vi "9871_EPICS_FPGA_Main.vi"() -> ()   [LabVIEW 2020]
uses:
  <vilib>/rvi/Emulation/niFpgaGetClockAttributes.vi
  <vilib>/rvi/Emulation/niFpgaSctlEmulationGetInTimedLoop.vi
  <vilib>/rvi/Emulation/niFpgaEmulationReportErrorSimple.vi
  <vilib>/rvi/interface/RandomDataEmulation/niFpgaRandomDataHandleErrors.vi
  <vilib>/rvi/eio/common/nirviEmuTemplateMethod_errors.vi
  <vilib>/rvi/Emulation/niFpgaCriticalErrorInLSC.vi
  <vilib>/rvi/eio/common/nirviEmuTemplatePropertySet_errors.vi
  <vilib>/rvi/DataTransferAndStorage/Container/XNode/niFpgaContainer.xnode
  <vilib>/rvi/interface/RandomDataEmulation/nirviRandomDataFpgaReadWriteTemplate.vi
  <vilib>/eio/EIOMethodNode/EIOMethodNode.xnode
  <vilib>/eio/EIOPropertyNode/EIOPropertyNode.xnode
  <vilib>/LabVIEW Targets/FPGA/cRIO/shared/nicrio_ModuleControls/nicrio_cRIO-9871_BaudRateEnum.ctl
  <vilib>/LabVIEW Targets/FPGA/cRIO/shared/nicrio_ModuleControls/nicrio_cRIO-9871_DataBitsEnum.ctl
  <vilib>/LabVIEW Targets/FPGA/cRIO/shared/nicrio_ModuleControls/nicrio_cRIO-9871_FlowControlEnum.ctl
  <vilib>/LabVIEW Targets/FPGA/cRIO/shared/nicrio_ModuleControls/nicrio_cRIO-9871_ParityEnum.ctl
  <vilib>/LabVIEW Targets/FPGA/cRIO/shared/nicrio_ModuleControls/nicrio_cRIO-9871_StopBitsEnum.ctl
  <vilib>/rvi/eio/common/nirviEmuTemplatePropertyGet_errors.vi
  <vilib>/rvi/eio/common/nirviEmuTemplatePropertyGet_noerrors.vi
  <vilib>/rvi/eio/common/nirviEmuTemplatePropertySet_noerrors.vi
panel:
  out "P3ReadError":errorcluster
  out "RX3FIFOTOCount":u32
  out "RX3ErrorCount":u32
  out "P4ReadError":errorcluster
  out "RX4FIFOTOCount":u32
  out "RX4ErrorCount":u32
  out "P2ReadError":errorcluster
  out "RX2FIFOTOCount":u32
  out "RX2ErrorCount":u32
  out "RX1FIFOTOCount":u32
  out "RX1ErrorCount":u32
  out "TXTOCount":u32
  out "TXErrorCount":u32
  out "P1ReadError":errorcluster
  out "WriteError":errorcluster
  # "WRITE"
  # "READ"
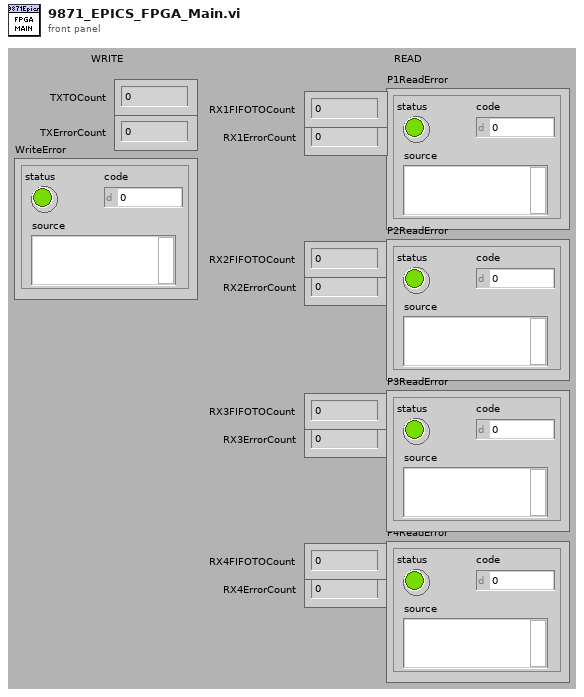
[diagram p1: front panel]
types:
  T1 = enum16{"TX Byte", "TX Clear", "Echo Request", "Parameter Change"}
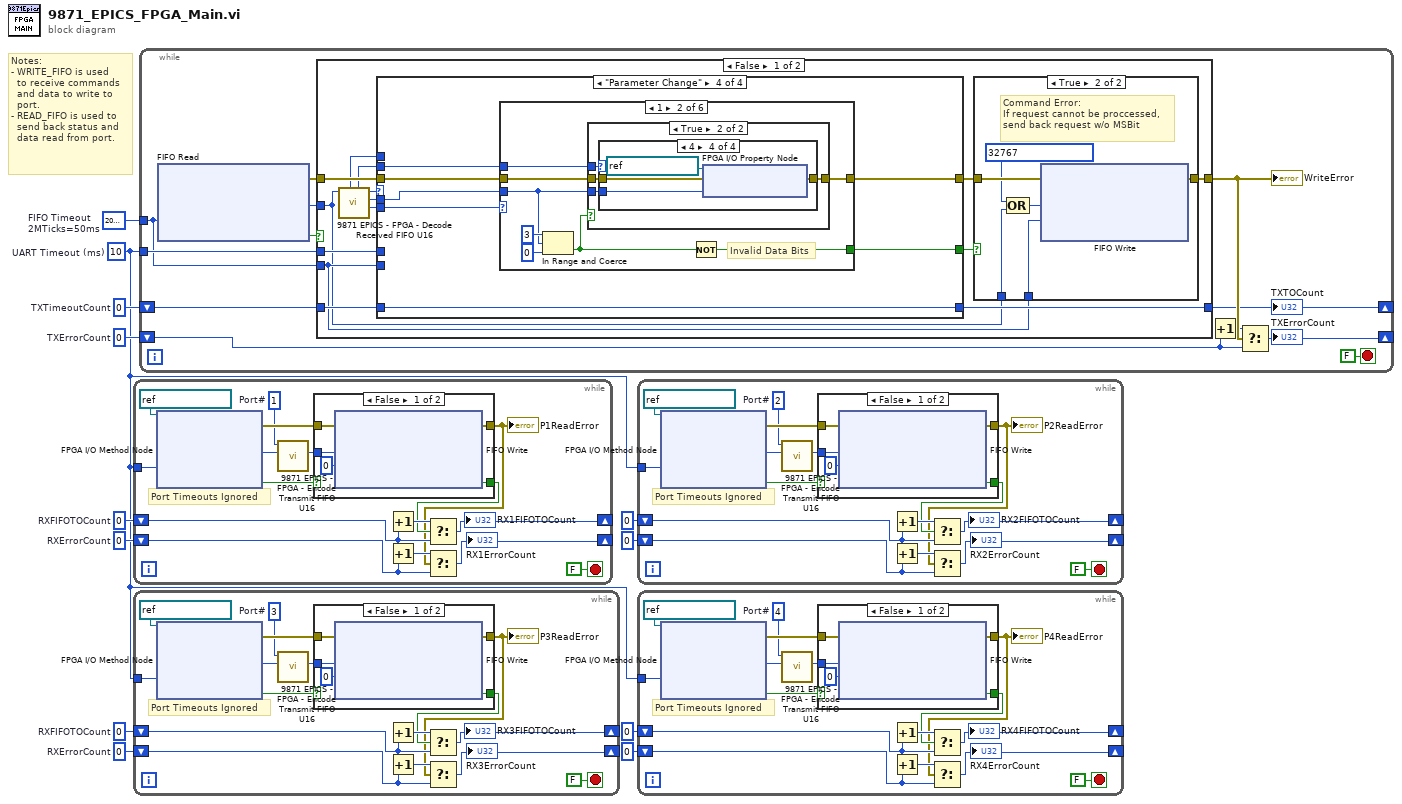
[diagram p0: block diagram]
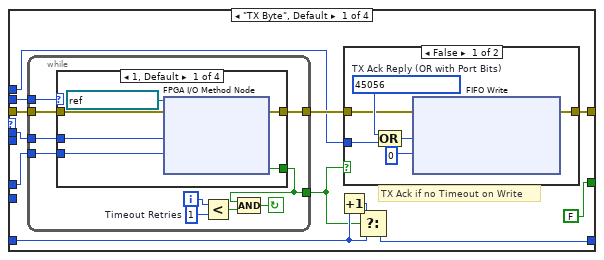
[diagram p6: hidden frame]
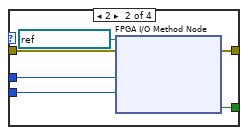
[diagram p8: hidden frame]
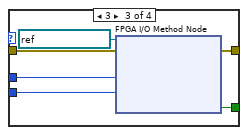
[diagram p9: hidden frame]
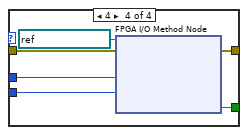
[diagram p10: hidden frame]
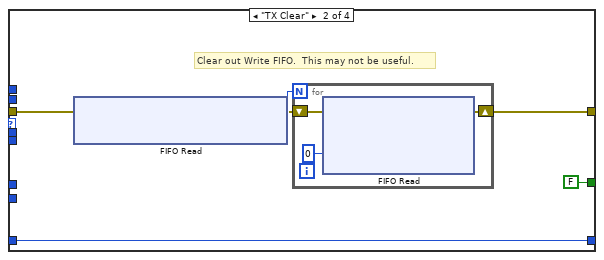
[diagram p11: hidden frame]
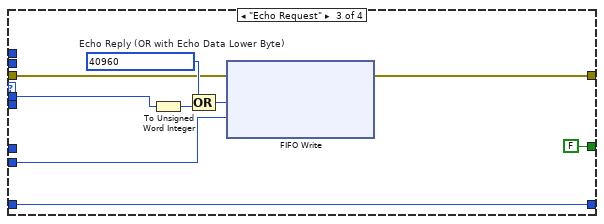
[diagram p12: hidden frame]
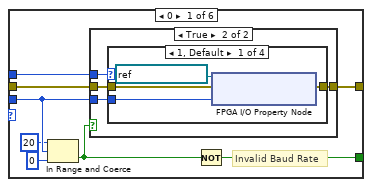
[diagram p13: hidden frame]
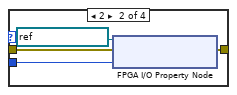
[diagram p15: hidden frame]
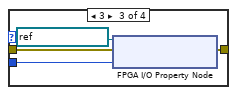
[diagram p16: hidden frame]
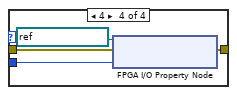
[diagram p17: hidden frame]
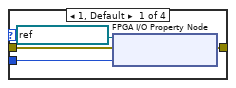
[diagram p19: hidden frame]
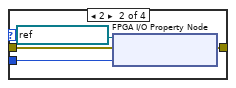
[diagram p20: hidden frame]
diagram:
  w3 = u32 0  # RXErrorCount
  w2 = u32 0  # RXFIFOTOCount
  w8 = u32 0  # RXErrorCount
  w9 = u32 0  # RXFIFOTOCount
  w10 = u32 0  # TXErrorCount
  w1 = 10  # UART Timeout (ms)
  w12 = 2000000  # FIFO Timeout 2MTicks=50ms
  w11 = u32 0  # TXTimeoutCount
  # "Notes:\n- WRITE_FIFO is used\n  to receive commands\n  and data to write to\n  port.\n- READ_FIFO is used to\n  send back status and\n  data read from port."
  n1 = while {
    tunnel: w1 -> [w26]
    shift-right: [w14] -> _
    shift-left: w9 -> [w18]
    shift-right: [w13] -> _
    shift-left: w8 -> [w15]
    stop <- FALSE stop-if-true
    w22 = u8 1  # Port#
    # "Port Timeouts Ignored"
    n2 = xnode "FPGA I/O Method Node"("FPGA I/O In"=refnum<k21> "Mod1\\Port1" ("cRIO I/O Device"), "Timeout (ms)"=w26) -> ("error out"=w24:errorcluster, "Data"=w23:u8, "Timed Out"=w25:bool)  [unwired: 1 in, 1 out]
    n3 = call "9871 EPICS - FPGA - Encode Transmit FIFO U16.vi"("Data Byte"=w23, "Port# (1-4)"=w22) -> ("U16 to Send to TX FIFO"=w21:u16)  [unwired: 9 in]
    n4 = case shown="False" w25 {
      tunnel: [w33 _] -> w19
      tunnel: w21 -> [w29 _]
      tunnel: [w31 w34] -> w16
      tunnel: w24 -> [w30 w34]
      frame False {
        n5 = xnode ("FIFO Write")("Element"=w29, "Timeout"=0, "error in (no error)"=w30) -> ("Timed Out?"=w33:bool, "error out"=w31:errorcluster)  [unwired: 1 in, 1 out]
      }
      frame True {
      }
    }
    "P1ReadError" <- w16
    n6 = Increment(x=w18) -> (x+1=w20:u32)
    n7 = Increment(x=w15) -> (x+1=w17:u32)
    n8 = Select(t=w20, s=w19, f=w18) -> (s? t:f=w14:u32)
    "RX1FIFOTOCount" <- w14
    n9 = Select(t=w17, s=w16, f=w15) -> (s? t:f=w13:u32)
    "RX1ErrorCount" <- w13
  }
  n10 = while {
    tunnel: w1 -> [w48]
    shift-right: [w36] -> _
    shift-left: w2 -> [w40]
    shift-right: [w35] -> _
    shift-left: w3 -> [w37]
    stop <- FALSE stop-if-true
    w44 = u8 3  # Port#
    # "Port Timeouts Ignored"
    n11 = xnode "FPGA I/O Method Node"("FPGA I/O In"=refnum<k21> "Mod1\\Port3" ("cRIO I/O Device"), "Timeout (ms)"=w48) -> ("error out"=w46:errorcluster, "Data"=w45:u8, "Timed Out"=w47:bool)  [unwired: 1 in, 1 out]
    n12 = call "9871 EPICS - FPGA - Encode Transmit FIFO U16.vi"("Data Byte"=w45, "Port# (1-4)"=w44) -> ("U16 to Send to TX FIFO"=w43:u16)  [unwired: 9 in]
    n13 = case shown="False" w47 {
      tunnel: [w55 _] -> w41
      tunnel: w43 -> [w51 _]
      tunnel: [w53 w56] -> w38
      tunnel: w46 -> [w52 w56]
      frame False {
        n14 = xnode ("FIFO Write")("Element"=w51, "Timeout"=0, "error in (no error)"=w52) -> ("Timed Out?"=w55:bool, "error out"=w53:errorcluster)  [unwired: 1 in, 1 out]
      }
      frame True {
      }
    }
    "P3ReadError" <- w38
    n15 = Increment(x=w40) -> (x+1=w42:u32)
    n16 = Increment(x=w37) -> (x+1=w39:u32)
    n17 = Select(t=w42, s=w41, f=w40) -> (s? t:f=w36:u32)
    "RX3FIFOTOCount" <- w36
    n18 = Select(t=w39, s=w38, f=w37) -> (s? t:f=w35:u32)
    "RX3ErrorCount" <- w35
  }
  n19 = while {
    shift-right: [w57] -> _
    shift-left: w11 -> [w64]
    tunnel: w12 -> [w62]
    tunnel: w1 -> [w63]
    shift-right: [w58] -> _
    shift-left: w10 -> [w59]
    stop <- FALSE stop-if-true
    n20 = xnode ("FIFO Read")("Timeout"=w62) -> ("Element"=w65:u16, "Timed Out?"=w66:bool, "error out"=w67:errorcluster)  [unwired: 2 in, 1 out]
    n21 = case shown="False" w66 {
      tunnel: [w72 w316] -> w61
      tunnel: w63 -> [w82 _]
      tunnel: w67 -> [w81 w316]
      tunnel: w65 -> [w70 _]
      tunnel: w64 -> [w78 w315]
      tunnel: [w77 w315] -> w57
      tunnel: w62 -> [w71 _]
      frame False {
        n22 = call "9871 EPICS - FPGA - Decode Received FIFO U16.vi"("U16"=w70) -> ("Parameter High Nibble Mid 4 bits  (xxNNNNxx xxxxxxxx)"=w74:u8, "Low Byte (xxxxxxxx NNNNNNNN)"=w79:u8, "Request Type"=w80:T1, "Port# (1-4)"=w76:u8, "Port Bits Only in U16"=w75:u16)  [unwired: 6 in]
        n23 = case shown="\"Parameter Change\"" w80 {
          tunnel: [w93 w144 w153 w162] -> w73
          tunnel: w82 -> [w101 _ _ _]
          tunnel: w81 -> [w98 w147 w154 w165]
          tunnel: w79 -> [w99 _ w159 w166]
          tunnel: w76 -> [w100 _ _ w163]
          tunnel: w78 -> [w96 w148 w160 w167]
          tunnel: [w97 w148 w160 w167] -> w77
          tunnel: w71 -> [_ _ w157 _]
          tunnel: w75 -> [w91 _ _ _]
          tunnel: w74 -> [_ _ _ w164]
          tunnel: [FALSE FALSE FALSE w161] -> w69
          frame "TX Byte", Default {
            # "TX Ack if no Timeout on Write"
            n24 = while {
              tunnel: w101 -> [w118]
              tunnel: [w112] -> w92
              tunnel: w100 -> [w117]
              tunnel: w99 -> [w116]
              tunnel: w98 -> [w111]
              tunnel: [w110] -> w94
              i -> [w115]
              stop <- w109 continue-if-true
              w114 = 1  # Timeout Retries
              n25 = case shown="1, Default" w117 {
                tunnel: w116 -> [w124 w130 w136 w142]
                tunnel: w118 -> [w123 w129 w135 w141]
                tunnel: [w122 w128 w134 w140] -> w112
                tunnel: w111 -> [w121 w127 w133 w139]
                tunnel: [w120 w126 w132 w138] -> w110
                frame 1, Default {
                  n26 = xnode "FPGA I/O Method Node"("error in"=w121, "FPGA I/O In"=refnum<k21> "Mod1\\Port1" ("cRIO I/O Device"), "Data"=w124, "Timeout (ms)"=w123) -> ("error out"=w120:errorcluster, "Timed Out"=w122:bool)  [unwired: 1 out]
                }
                frame 2 {
                  n27 = xnode "FPGA I/O Method Node"("error in"=w127, "FPGA I/O In"=refnum<k21> "Mod1\\Port2" ("cRIO I/O Device"), "Data"=w130, "Timeout (ms)"=w129) -> ("error out"=w126:errorcluster, "Timed Out"=w128:bool)  [unwired: 1 out]
                }
                frame 3 {
                  n28 = xnode "FPGA I/O Method Node"("error in"=w133, "FPGA I/O In"=refnum<k21> "Mod1\\Port3" ("cRIO I/O Device"), "Data"=w136, "Timeout (ms)"=w135) -> ("error out"=w132:errorcluster, "Timed Out"=w134:bool)  [unwired: 1 out]
                }
                frame 4 {
                  n29 = xnode "FPGA I/O Method Node"("error in"=w139, "FPGA I/O In"=refnum<k21> "Mod1\\Port4" ("cRIO I/O Device"), "Data"=w142, "Timeout (ms)"=w141) -> ("error out"=w138:errorcluster, "Timed Out"=w140:bool)  [unwired: 1 out]
                }
              }
              n30 = Less?(x=w115, y=w114) -> (x < y?=w113:bool)
              n31 = Compound Arithmetic op=AND(w112, w113) -> (w109:bool)
            }
            n32 = Increment(x=w96) -> (x+1=w95:u32)
            n33 = case shown="False" w92 {
              tunnel: w94 -> [w105 w108]
              tunnel: [w104 w108] -> w93
              tunnel: w91 -> [w103 _]
              frame False {
                w106 = u16 45056  # TX Ack Reply (OR with Port Bits)
                n34 = Compound Arithmetic op=OR(w106, w103) -> (w107:u16)
                n35 = xnode ("FIFO Write")("Element"=w107, "Timeout"=0, "error in (no error)"=w105) -> ("error out"=w104:errorcluster)  [unwired: 1 in, 2 out]
              }
              frame True {
              }
            }
            n36 = Select(t=w95, s=w92, f=w96) -> (s? t:f=w97:u32)
          }
          frame "TX Clear" {
            # "Clear out Write FIFO.  This may not be useful."
            n37 = xnode ("FIFO Read")("error in (no error)"=w147) -> ("Number of Elements to Read"=w146:u32, "error out"=w145:errorcluster)  [unwired: 1 in, 1 out]
            n38 = for {
              N: w146 -> [_]
              shift-right: [w150] -> w144
              shift-left: w145 -> [w151]
              n39 = xnode ("FIFO Read")("Timeout"=0, "error in (no error)"=w151) -> ("error out"=w150:errorcluster)  [unwired: 1 in, 3 out]
            }
          }
          frame "Echo Request" {
            w156 = u16 40960  # Echo Reply (OR with Echo Data Lower Byte)
            n40 = To Unsigned Word Integer(number=w159) -> (unsigned 16bit integer=w158:u16)
            n41 = Compound Arithmetic op=OR(w156, w158) -> (w155:u16)
            n42 = xnode ("FIFO Write")("Element"=w155, "Timeout"=w157, "error in (no error)"=w154) -> ("error out"=w153:errorcluster)  [unwired: 1 in, 2 out]
          }
          frame "Parameter Change" {
            n43 = case shown="1" w164 {
              tunnel: w166 -> [w172 w199 w228 w256 w286 _]
              tunnel: w165 -> [w175 w204 w233 w262 w291 w314]
              tunnel: [w174 w203 w232 w261 w290 w314] -> w162
              tunnel: [w168 w198 w227 w257 w285 w313] -> w161
              tunnel: w163 -> [w173 w202 w231 w260 w289 _]
              frame 0 {
                # "Invalid Baud Rate"
                n44 = In Range and Coerce(upper limit=u8 20, x=w172, lower limit=u8 0) -> (In Range?=w169:bool)  [unwired: 1 out]
                n45 = case shown="True" w169 {
                  tunnel: w175 -> [w176 w180]
                  tunnel: [w176 w179] -> w174
                  tunnel: w173 -> [_ w178]
                  tunnel: w172 -> [_ w177]
                  frame False {
                  }
                  frame True {
                    n46 = case shown="1, Default" w178 {
                      tunnel: w177 -> [w183 w187 w191 w195]
                      tunnel: w180 -> [w182 w186 w190 w194]
                      tunnel: [w181 w185 w189 w193] -> w179
                      frame 1, Default {
                        n47 = xnode "FPGA I/O Property Node"("error in"=w182, "FPGA I/O In"=refnum<k21> "Mod1\\Port1" ("cRIO I/O Device"), "Baud Rate"=w183) -> ("error out"=w181:errorcluster)  [unwired: 1 out]
                      }
                      frame 2 {
                        n48 = xnode "FPGA I/O Property Node"("error in"=w186, "FPGA I/O In"=refnum<k21> "Mod1\\Port2" ("cRIO I/O Device"), "Baud Rate"=w187) -> ("error out"=w185:errorcluster)  [unwired: 1 out]
                      }
                      frame 3 {
                        n49 = xnode "FPGA I/O Property Node"("error in"=w190, "FPGA I/O In"=refnum<k21> "Mod1\\Port3" ("cRIO I/O Device"), "Baud Rate"=w191) -> ("error out"=w189:errorcluster)  [unwired: 1 out]
                      }
                      frame 4 {
                        n50 = xnode "FPGA I/O Property Node"("error in"=w194, "FPGA I/O In"=refnum<k21> "Mod1\\Port4" ("cRIO I/O Device"), "Baud Rate"=w195) -> ("error out"=w193:errorcluster)  [unwired: 1 out]
                      }
                    }
                  }
                }
                n51 = Not(x=w169) -> (.not. x?=w168:bool)
              }
              frame 1 {
                # "Invalid Data Bits"
                n52 = In Range and Coerce(upper limit=u8 3, x=w199, lower limit=u8 0) -> (In Range?=w197:bool)  [unwired: 1 out]
                n53 = case shown="True" w197 {
                  tunnel: w204 -> [w205 w209]
                  tunnel: [w205 w208] -> w203
                  tunnel: w202 -> [_ w207]
                  tunnel: w199 -> [_ w206]
                  frame False {
                  }
                  frame True {
                    n54 = case shown="4" w207 {
                      tunnel: w206 -> [w212 w216 w220 w224]
                      tunnel: w209 -> [w211 w215 w219 w223]
                      tunnel: [w210 w214 w218 w222] -> w208
                      frame 1, Default {
                        n55 = xnode "FPGA I/O Property Node"("error in"=w211, "FPGA I/O In"=refnum<k21> "Mod1\\Port1" ("cRIO I/O Device"), "Data Bits"=w212) -> ("error out"=w210:errorcluster)  [unwired: 1 out]
                      }
                      frame 2 {
                        n56 = xnode "FPGA I/O Property Node"("error in"=w215, "FPGA I/O In"=refnum<k21> "Mod1\\Port2" ("cRIO I/O Device"), "Data Bits"=w216) -> ("error out"=w214:errorcluster)  [unwired: 1 out]
                      }
                      frame 3 {
                        n57 = xnode "FPGA I/O Property Node"("error in"=w219, "FPGA I/O In"=refnum<k21> "Mod1\\Port3" ("cRIO I/O Device"), "Data Bits"=w220) -> ("error out"=w218:errorcluster)  [unwired: 1 out]
                      }
                      frame 4 {
                        n58 = xnode "FPGA I/O Property Node"("error in"=w223, "FPGA I/O In"=refnum<k21> "Mod1\\Port4" ("cRIO I/O Device"), "Data Bits"=w224) -> ("error out"=w222:errorcluster)  [unwired: 1 out]
                      }
                    }
                  }
                }
                n59 = Not(x=w197) -> (.not. x?=w198:bool)
              }
              frame 2 {
                # "Invalid Flow Control"
                n60 = In Range and Coerce(upper limit=u8 2, x=w228, lower limit=u8 0) -> (In Range?=w226:bool)  [unwired: 1 out]
                n61 = case shown="True" w226 {
                  tunnel: w233 -> [w234 w238]
                  tunnel: [w234 w237] -> w232
                  tunnel: w231 -> [_ w236]
                  tunnel: w228 -> [_ w235]
                  frame False {
                  }
                  frame True {
                    n62 = case shown="1, Default" w236 {
                      tunnel: w235 -> [w241 w245 w249 w253]
                      tunnel: w238 -> [w240 w244 w248 w252]
                      tunnel: [w239 w243 w247 w251] -> w237
                      frame 1, Default {
                        n63 = xnode "FPGA I/O Property Node"("error in"=w240, "FPGA I/O In"=refnum<k21> "Mod1\\Port1" ("cRIO I/O Device"), "Flow Control"=w241) -> ("error out"=w239:errorcluster)  [unwired: 1 out]
                      }
                      frame 2 {
                        n64 = xnode "FPGA I/O Property Node"("error in"=w244, "FPGA I/O In"=refnum<k21> "Mod1\\Port2" ("cRIO I/O Device"), "Flow Control"=w245) -> ("error out"=w243:errorcluster)  [unwired: 1 out]
                      }
                      frame 3 {
                        n65 = xnode "FPGA I/O Property Node"("error in"=w248, "FPGA I/O In"=refnum<k21> "Mod1\\Port3" ("cRIO I/O Device"), "Flow Control"=w249) -> ("error out"=w247:errorcluster)  [unwired: 1 out]
                      }
                      frame 4 {
                        n66 = xnode "FPGA I/O Property Node"("error in"=w252, "FPGA I/O In"=refnum<k21> "Mod1\\Port4" ("cRIO I/O Device"), "Flow Control"=w253) -> ("error out"=w251:errorcluster)  [unwired: 1 out]
                      }
                    }
                  }
                }
                n67 = Not(x=w226) -> (.not. x?=w227:bool)
              }
              frame 3 {
                # "Invalid Parity"
                n68 = In Range and Coerce(upper limit=u8 4, x=w256, lower limit=u8 0) -> (In Range?=w255:bool)  [unwired: 1 out]
                n69 = case shown="True" w255 {
                  tunnel: w262 -> [w263 w267]
                  tunnel: [w263 w266] -> w261
                  tunnel: w260 -> [_ w265]
                  tunnel: w256 -> [_ w264]
                  frame False {
                  }
                  frame True {
                    n70 = case shown="4" w265 {
                      tunnel: w264 -> [w270 w274 w278 w282]
                      tunnel: w267 -> [w269 w273 w277 w281]
                      tunnel: [w268 w272 w276 w280] -> w266
                      frame 1, Default {
                        n71 = xnode "FPGA I/O Property Node"("error in"=w269, "FPGA I/O In"=refnum<k21> "Mod1\\Port1" ("cRIO I/O Device"), "Parity"=w270) -> ("error out"=w268:errorcluster)  [unwired: 1 out]
                      }
                      frame 2 {
                        n72 = xnode "FPGA I/O Property Node"("error in"=w273, "FPGA I/O In"=refnum<k21> "Mod1\\Port2" ("cRIO I/O Device"), "Parity"=w274) -> ("error out"=w272:errorcluster)  [unwired: 1 out]
                      }
                      frame 3 {
                        n73 = xnode "FPGA I/O Property Node"("error in"=w277, "FPGA I/O In"=refnum<k21> "Mod1\\Port3" ("cRIO I/O Device"), "Parity"=w278) -> ("error out"=w276:errorcluster)  [unwired: 1 out]
                      }
                      frame 4 {
                        n74 = xnode "FPGA I/O Property Node"("error in"=w281, "FPGA I/O In"=refnum<k21> "Mod1\\Port4" ("cRIO I/O Device"), "Parity"=w282) -> ("error out"=w280:errorcluster)  [unwired: 1 out]
                      }
                    }
                  }
                }
                n75 = Not(x=w255) -> (.not. x?=w257:bool)
              }
              frame 4 {
                # "Invalid Stop Bits"
                n76 = In Range and Coerce(upper limit=u8 2, x=w286, lower limit=u8 0) -> (In Range?=w284:bool)  [unwired: 1 out]
                n77 = case shown="True" w284 {
                  tunnel: w291 -> [w292 w296]
                  tunnel: [w292 w295] -> w290
                  tunnel: w289 -> [_ w294]
                  tunnel: w286 -> [_ w293]
                  frame False {
                  }
                  frame True {
                    n78 = case shown="4" w294 {
                      tunnel: w293 -> [w299 w303 w307 w311]
                      tunnel: w296 -> [w298 w302 w306 w310]
                      tunnel: [w297 w301 w305 w309] -> w295
                      frame 1, Default {
                        n79 = xnode "FPGA I/O Property Node"("error in"=w298, "FPGA I/O In"=refnum<k21> "Mod1\\Port1" ("cRIO I/O Device"), "Stop Bits"=w299) -> ("error out"=w297:errorcluster)  [unwired: 1 out]
                      }
                      frame 2 {
                        n80 = xnode "FPGA I/O Property Node"("error in"=w302, "FPGA I/O In"=refnum<k21> "Mod1\\Port2" ("cRIO I/O Device"), "Stop Bits"=w303) -> ("error out"=w301:errorcluster)  [unwired: 1 out]
                      }
                      frame 3 {
                        n81 = xnode "FPGA I/O Property Node"("error in"=w306, "FPGA I/O In"=refnum<k21> "Mod1\\Port3" ("cRIO I/O Device"), "Stop Bits"=w307) -> ("error out"=w305:errorcluster)  [unwired: 1 out]
                      }
                      frame 4 {
                        n82 = xnode "FPGA I/O Property Node"("error in"=w310, "FPGA I/O In"=refnum<k21> "Mod1\\Port4" ("cRIO I/O Device"), "Stop Bits"=w311) -> ("error out"=w309:errorcluster)  [unwired: 1 out]
                      }
                    }
                  }
                }
                n83 = Not(x=w284) -> (.not. x?=w285:bool)
              }
              frame 5.. {
                w313 = TRUE  # Invalid UART Parameter ID
              }
            }
          }
        }
        n84 = case shown="True" w69 {
          tunnel: w73 -> [w83 w88]
          tunnel: [w83 w87] -> w72
          tunnel: w71 -> [_ w86]
          tunnel: w70 -> [_ w85]
          frame False {
          }
          frame True {
            # "Command Error:\nIf request cannot be proccessed,\nsend back request w/o MSBit"
            n85 = Compound Arithmetic op=OR(u16 32767, w85) -> (w89:u16)
            n86 = xnode ("FIFO Write")("Element"=w89, "Timeout"=w86, "error in (no error)"=w88) -> ("error out"=w87:errorcluster)  [unwired: 1 in, 2 out]
          }
        }
      }
      frame True {
      }
    }
    "WriteError" <- w61
    "TXTOCount" <- w57
    n87 = Increment(x=w59) -> (x+1=w60:u32)
    n88 = Select(t=w60, s=w61, f=w59) -> (s? t:f=w58:u32)
    "TXErrorCount" <- w58
  }
  n89 = while {
    tunnel: w1 -> [w330]
    shift-right: [w318] -> _
    shift-left: u32 0 ("RXFIFOTOCount") -> [w322]
    shift-right: [w317] -> _
    shift-left: u32 0 ("RXErrorCount") -> [w319]
    stop <- FALSE stop-if-true
    w326 = u8 2  # Port#
    # "Port Timeouts Ignored"
    n90 = xnode "FPGA I/O Method Node"("FPGA I/O In"=refnum<k21> "Mod1\\Port2" ("cRIO I/O Device"), "Timeout (ms)"=w330) -> ("error out"=w328:errorcluster, "Data"=w327:u8, "Timed Out"=w329:bool)  [unwired: 1 in, 1 out]
    n91 = call "9871 EPICS - FPGA - Encode Transmit FIFO U16.vi"("Data Byte"=w327, "Port# (1-4)"=w326) -> ("U16 to Send to TX FIFO"=w325:u16)  [unwired: 9 in]
    n92 = case shown="False" w329 {
      tunnel: [w337 _] -> w323
      tunnel: w325 -> [w333 _]
      tunnel: [w335 w338] -> w320
      tunnel: w328 -> [w334 w338]
      frame False {
        n93 = xnode ("FIFO Write")("Element"=w333, "Timeout"=0, "error in (no error)"=w334) -> ("Timed Out?"=w337:bool, "error out"=w335:errorcluster)  [unwired: 1 in, 1 out]
      }
      frame True {
      }
    }
    "P2ReadError" <- w320
    n94 = Increment(x=w322) -> (x+1=w324:u32)
    n95 = Increment(x=w319) -> (x+1=w321:u32)
    n96 = Select(t=w324, s=w323, f=w322) -> (s? t:f=w318:u32)
    "RX2FIFOTOCount" <- w318
    n97 = Select(t=w321, s=w320, f=w319) -> (s? t:f=w317:u32)
    "RX2ErrorCount" <- w317
  }
  n98 = while {
    tunnel: w1 -> [w352]
    shift-right: [w340] -> _
    shift-left: u32 0 ("RXFIFOTOCount") -> [w344]
    shift-right: [w339] -> _
    shift-left: u32 0 ("RXErrorCount") -> [w341]
    stop <- FALSE stop-if-true
    w348 = u8 4  # Port#
    # "Port Timeouts Ignored"
    n99 = xnode "FPGA I/O Method Node"("FPGA I/O In"=refnum<k21> "Mod1\\Port4" ("cRIO I/O Device"), "Timeout (ms)"=w352) -> ("error out"=w350:errorcluster, "Data"=w349:u8, "Timed Out"=w351:bool)  [unwired: 1 in, 1 out]
    n100 = call "9871 EPICS - FPGA - Encode Transmit FIFO U16.vi"("Data Byte"=w349, "Port# (1-4)"=w348) -> ("U16 to Send to TX FIFO"=w347:u16)  [unwired: 9 in]
    n101 = case shown="False" w351 {
      tunnel: [w359 _] -> w345
      tunnel: w347 -> [w355 _]
      tunnel: [w357 w360] -> w342
      tunnel: w350 -> [w356 w360]
      frame False {
        n102 = xnode ("FIFO Write")("Element"=w355, "Timeout"=0, "error in (no error)"=w356) -> ("Timed Out?"=w359:bool, "error out"=w357:errorcluster)  [unwired: 1 in, 1 out]
      }
      frame True {
      }
    }
    "P4ReadError" <- w342
    n103 = Increment(x=w344) -> (x+1=w346:u32)
    n104 = Increment(x=w341) -> (x+1=w343:u32)
    n105 = Select(t=w346, s=w345, f=w344) -> (s? t:f=w340:u32)
    "RX4FIFOTOCount" <- w340
    n106 = Select(t=w343, s=w342, f=w341) -> (s? t:f=w339:u32)
    "RX4ErrorCount" <- w339
  }
